vi "Receptor PSK.vi"() -> ()   [LabVIEW 2016]
uses:
  <vilib>/addons/Modulation/Analog/support/mod_Set Error Source.vi
  <vilib>/addons/Modulation/Analog/support/Validators/mod_Fractional Resample Validate.vi
  <vilib>/addons/Modulation/Analog/support/Validators/mod_Check Flush State.vi
  <vilib>/addons/Modulation/Analog/support/mod_FractionalResampler.vi
  <vilib>/addons/Modulation/Analog/support/mod_Integer Rate Interpolation.vi
  <vilib>/addons/Modulation/Analog/support/Validators/mod_Validate Complex Waveform.vi
  <vilib>/addons/Modulation/Analog/support/mod_PerformResampling.vi
  <vilib>/addons/Modulation/Analog/support/Validators/mod_WFErrorHandler.vi
  <vilib>/addons/Modulation/Digital/Support/Common/Validators/mod_Generate Filter Coefficients Validate.vi
  <vilib>/addons/Modulation/Digital/General/subVIs/mod_Generate Filter Coefficients.vi
  <instrlib>/niUSRP/niUSRP Fetch Rx Data (CDB Cluster).vi
  <vilib>/addons/Modulation/Digital/General/MT Generate PSK System Parameters(M).vi
  <vilib>/Utility/error.llb/Error Cluster From Error Code.vi
  <vilib>/addons/Modulation/Analog/support/mod_Resampling Factors.vi
  <vilib>/addons/Modulation/Analog/support/mod_ResamplingFilter.vi
  <vilib>/addons/Modulation/Analog/support/mod_Generate Integer Interpolation Filter.vi
  <instrlib>/niUSRP/niUSRP Fetch Rx Data (CDB WDT).vi
  <vilib>/measure/maspectr.llb/FFT Spectrum (Mag-Phase) for 1 Chan (CDB).vi
  <vilib>/addons/Modulation/niDMT.lvlib
  <vilib>/addons/Modulation/niAMT.lvlib
  <vilib>/measure/NI_MAPro.lvlib
panel:
  out "Symbol rate":dbl
  out "output bit stream":i8[](array[numeric])
  out "Magnitude Spectrum":cluster{"f0":dbl, "df":dbl, "magnitude":dbl[]}(graph)={"f0"=-100000.0, "df"=20.0, "magnitude"=[]}
  out "Acquired Signal":waveform(dbl)[](graph)
  out "Frame Size [samples]":i64=20000
  in  "Acq Duration [sec]":dbl=0.01 format="%#.6p"
  in  "autoscale":bool
  out "Constellation Graph":T1(graph)
  in  "stop":bool
  out "measurements":T2={"frequency offset (Hz)"=-11.93165072236316, "frequency drift (Hz)"=0.08770196207837619, "phase offset (deg)"=52.673364140832604} {"phase offset (deg)" format="%.2f"; "frequency drift (Hz)" format="%.2f"; "frequency offset (Hz)" format="%.2f"}
  in  "filter parameters":T3={"Alpha"=0.5, "Filter Length"=6, "TX Filter"=enum."Root Raised Cos"} {"Alpha" format="%.2f"}
  out "Gain [dB] (actual)":dbl=12.0 format="%#.6p"
  out "Carrier Frequency \n[Hz] (actual)":dbl=915000000.0 format="%#.6p"
  out "IQ Sampling\nRate [S/sec] (actual)":dbl=500000.0 format="%#.6p"
  in  "Active Antenna":string(combo)="RX1"
  in  "Gain [dB]":dbl=12.0 format="%#.6p"
  in  "Carrier\nFrequency [Hz]":dbl=915000000.0 format="%#.6p"
  in  "IQ Sampling\nRate [S/sec]":dbl=500000.0 format="%#.6p"
  out "session handle out":refnum<k15>
  in  "error in (no error)":errorcluster
  in  "device names":refnum<k15>
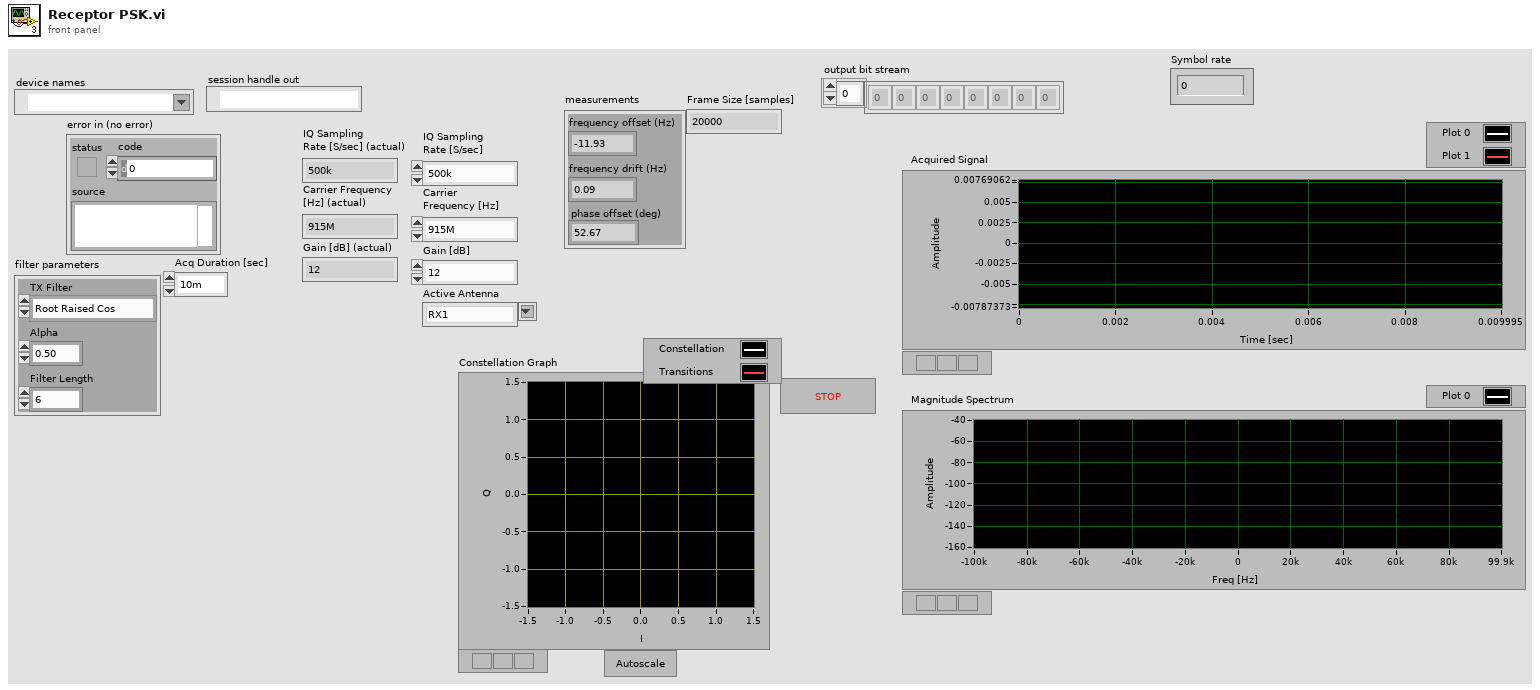
[diagram p1: front panel]
types:
  T1 = cluster{"Decimated Array":dbl[], "Decimated Array":dbl[]}[]
  T2 = cluster{"frequency offset (Hz)":dbl, "frequency drift (Hz)":dbl, "phase offset (deg)":dbl}
  T3 = cluster{"Alpha":dbl, "Filter Length":i32, "TX Filter":enum16{"none", "Raised Cosine", "Root Raised Cos", "Gaussian"}}
  T4 = enum16{"FSK", "PSK", "QAM", "MSK", "PAM", "ASK", "CPM"}
  T5 = enum16{"none", "Raised Cosine", "Root Raised Cos", "Gaussian"}
  T6 = cluster{"samples per symbol (16)":i32, "symbol map":cdb[], "differential PSK":enum16{"disable", "enable"}, "PSK type":u16}
  T7 = cluster{"dB On (F)":bool, "unwrap phase (F)":bool, "convert to degree (F)":bool}
  T8 = typedef "niAMT.lvlib/Complex Data Waveform.ctl" = cluster{"t0":dbl, "dt":dbl, "Y":cdb[]}
  T9 = cluster{"constellation":dbl[], "oversampled data":dbl[]}[]
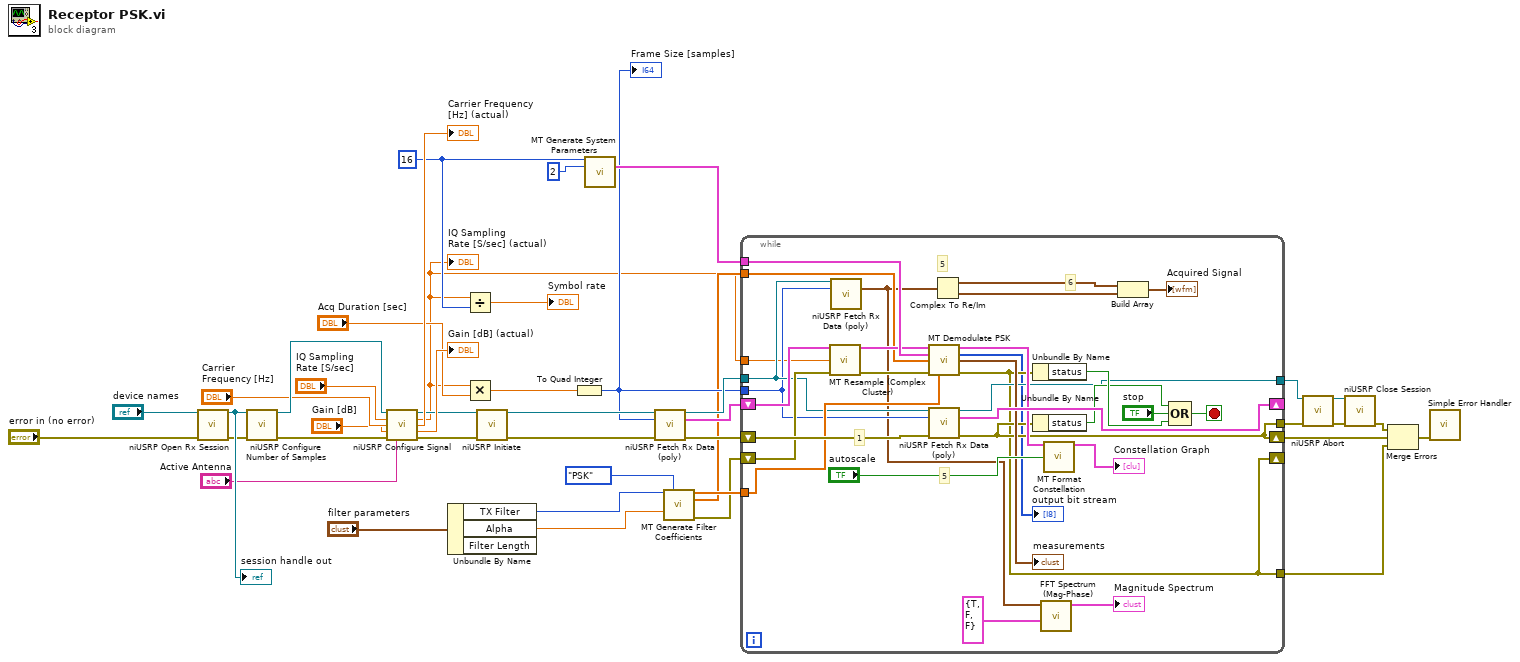
[diagram p0: block diagram]
diagram:
  w2 = 16 ("samples per symbol (16)")
  n1 = call <instrlib>:"niUSRP Open Rx Session.vi"("device names"="device names", "error in (no error)"="error in (no error)") -> ("session handle out"=w40:refnum<k15>, "error out"=w39:errorcluster)  [unwired: 12 in]
  "session handle out" <- w40
  n2 = call <instrlib>:"niUSRP Configure Number of Samples.vi"("session handle"=w40, "error in (no error)"=w39) -> ("session handle out"=w38:refnum<k15>, "error out"=w33:errorcluster)  [unwired: 12 in]
  n3 = call <instrlib>:"niUSRP Configure Signal.vi"("session handle"=w38, "IQ rate"="IQ Sampling\nRate [S/sec]", "carrier frequency"="Carrier\nFrequency [Hz]", "gain"="Gain [dB]", "error in (no error)"=w33, "active antenna"="Active Antenna") -> ("session handle out"=w30:refnum<k15>, "coerced IQ rate"=w1:dbl, "coerced carrier frequency"=→"Carrier Frequency \n[Hz] (actual)":dbl, "coerced gain"=→"Gain [dB] (actual)":dbl, "error out"=w29:errorcluster)  [unwired: 5 in]
  "IQ Sampling\nRate [S/sec] (actual)" <- w1
  n4 = Unbundle By Name("filter parameters") -> ("TX Filter"=w23:T5, "Alpha"=w24:dbl)  [unwired: 1 out]
  n5 = Divide(x=w1, y=w2) -> (x/y=→"Symbol rate":dbl)
  n6 = Multiply(x=w1, y="Acq Duration [sec]") -> (x*y=w15:dbl)
  n7 = call <instrlib>:"niUSRP Initiate.vi"("session handle"=w30, "error in (no error)"=w29) -> ("session handle out"=w28:refnum<k15>, "error out"=w27:errorcluster)  [unwired: 12 in]
  n8 = To Quad Integer(1:w15) -> (0:w14:i64)
  "Frame Size [samples]" <- w14
  n9 = call-poly <vilib>:"MT Generate System Parameters.vi"("samples per symbol (16)"=w2, "M-PSK (4)"=2) -> ("PSK system parameters"=w17:T6)  [unwired: 11 in, 2 out]
  n10 = call-poly <instrlib>:"niUSRP Fetch Rx Data (poly).vi"("session handle"=w28, "number of samples"=w14, "error in (no error)"=w27) -> ("session handle out"=w21:refnum<k15>, "data"=w19:cluster{"t0":dbl, "dt":dbl, "Y":cdb[]}, "error out"=w20:errorcluster)  [unwired: 9 in, 1 out]
  n11 = call <vilib>:"MT Generate Filter Coefficients.vi"("pulse shaping filter (none)"=w23, "modulation type"=T4."PSK", "filter parameter"=w24) -> ("pulse shaping filter coefficients"=w18:dbl[], "matched filter coefficients"=w4:dbl[], "error out"=w16:errorcluster)  [unwired: 10 in]
  n12 = while {
    tunnel: w21 -> [w52]
    shift-right: [w56] -> w8
    shift-left: w20 -> [w72]
    shift-right: [w71] -> _
    shift-left: w19 -> [w68]
    tunnel: w18 -> [w70]
    tunnel: w17 -> [w69]
    shift-right: [w54] -> _
    shift-left: w16 -> [w67]
    tunnel: w14 -> [w51]
    tunnel: [w56] -> w7
    tunnel: [w55] -> w6
    tunnel: [w54] -> w5
    tunnel: w4 -> [w53]
    tunnel: w1 -> [w43]
    stop <- w63 stop-if-true
    # "6"
    # "5"
    # "5"
    # "1"
    n13 = call <vilib>:"MT Resample (Complex Cluster).vi"("input complex waveform"=w68, "desired sample rate (Hz)"=w43, "error in (no error)"=w67) -> ("output complex waveform"=w65:T8, "error out"=w66:errorcluster)  [unwired: 11 in]
    n14 = call-poly <instrlib>:"niUSRP Fetch Rx Data (poly).vi"("session handle"=w52, "number of samples"=w51) -> ("data"=w45:waveform(cdb))  [unwired: 10 in, 3 out]
    n15 = call <vilib>:"MT Demodulate PSK.vi"("input complex waveform"=w65, "PSK system parameters"=w69, "matched filter coefficients"=w53, "error in (no error)"=w66, "pulse shaping filter coefficients"=w70) -> ("recovered complex waveform"=w58:T8, "output bit stream"=→"output bit stream":i8[], "measurements"=→"measurements":T2, "error out"=w54:errorcluster)  [unwired: 6 in, 1 out]
    n16 = call-poly <instrlib>:"niUSRP Fetch Rx Data (poly).vi"("session handle"=w52, "number of samples"=w51, "error in (no error)"=w72) -> ("session handle out"=w55:refnum<k15>, "data"=w71:cluster{"t0":dbl, "dt":dbl, "Y":cdb[]}, "error out"=w56:errorcluster)  [unwired: 9 in, 1 out]
    n17 = Complex To Re/Im(x + iy=w45) -> (x=w48:waveform(dbl), y=w47:waveform(dbl))
    n18 = Unbundle By Name(w54) -> ("status"=w60:bool)
    n19 = Unbundle By Name(w56) -> ("status"=w59:bool)
    n20 = call-poly <vilib>:"FFT Spectrum (Mag-Phase).vi"("view"=T7 {"dB On (F)"=TRUE, "unwrap phase (F)"=FALSE, "convert to degree (F)"=FALSE}, "time signal"=w45) -> ("magnitude"=→"Magnitude Spectrum":cluster{"f0":dbl, "df":dbl, "magnitude":dbl[]})  [unwired: 5 in, 4 out]
    n21 = call <vilib>:"MT Format Constellation.vi"("waveform"=w58, "autoscale"="autoscale") -> ("constellation graph"=→"Constellation Graph":T9)  [unwired: 12 in, 1 out]
    n22 = Build Array(w48, w47) -> (→"Acquired Signal":waveform(dbl)[])
    n23 = Compound Arithmetic op=OR(w59, "stop", w60) -> (w63:bool)
  }
  n24 = call <instrlib>:"niUSRP Abort.vi"("session handle"=w6, "error in (no error)"=w7) -> ("session handle out"=w11:refnum<k15>, "error out"=w10:errorcluster)  [unwired: 12 in]
  n25 = call <instrlib>:"niUSRP Close Session.vi"("session handle"=w11, "error in (no error)"=w10) -> ("error out"=w9:errorcluster)  [unwired: 13 in]
  n26 = Merge Errors(w9, w8, w5) -> (w12:errorcluster)
  n27 = call <vilib>:"Simple Error Handler.vi"("error in (no error)"=w12) -> ()  [unwired: 4 in, 5 out]
